vi "1A Helper - GPS Mode Parser.vi"(6 "GPS Mode (Char)":string) -> (2 "GPS Mode (Description)":string)   [LabVIEW 2013]
doc: "A simple parser to interpret single-character GPS Mode data into full descriptive strings."
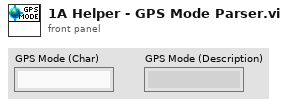
[diagram p1: front panel]
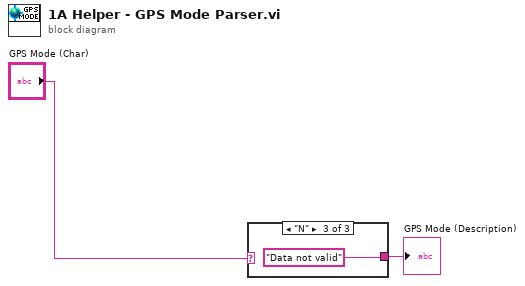
[diagram p0: block diagram]
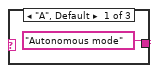
[diagram p2: hidden frame]
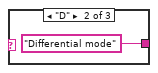
[diagram p3: hidden frame]
diagram:
  n1 = case shown="\"N\"" "GPS Mode (Char)" {
    tunnel: ["Autonomous mode" "Differential mode" "Data not valid"] -> w2
    frame "A", Default {
    }
    frame "D" {
    }
    frame "N" {
    }
  }
  "GPS Mode (Description)" <- w2
